vi "(Riemann) Zeta Function.vi"(3 "x":cdb) -> (1 "z(x)":cdb)   [LabVIEW 2014, in "NI_Gmath.lvlib"]
doc: "Computes the zeta function."
uses:
  NI_Gmath.lvlib
  lvanlys.dll
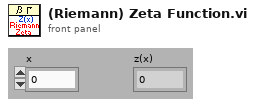
[diagram p1: front panel]
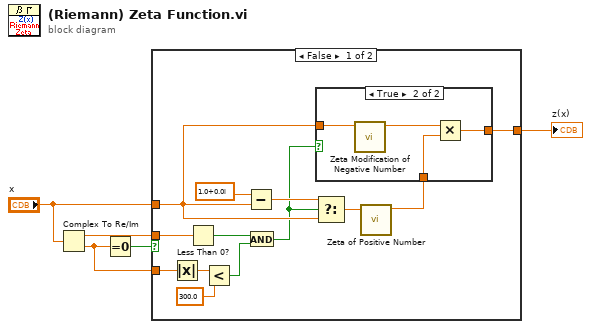
[diagram p0: block diagram]
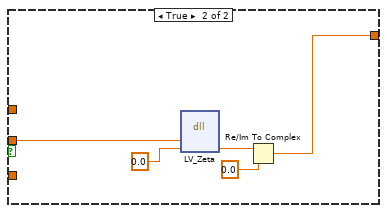
[diagram p3: hidden frame]
diagram:
  n1 = Complex To Re/Im(x + iy="x") -> (x=w5:dbl, y=w3:dbl)
  n2 = Equal To 0?(x=w3) -> (x = 0?=w4:bool)
  n3 = case shown="False" w4 {
    tunnel: "x" -> [w17 _]
    tunnel: w5 -> [w15 w28]
    tunnel: [w16 w25] -> w1
    tunnel: w3 -> [w11 _]
    frame False {
      n4 = Absolute Value(x=w11) -> (abs(x)=w10:dbl)
      n5 = Less Than 0?(x=w15) -> (x < 0?=w7:bool)
      n6 = Less?(x=w10, y=300.0) -> (x < y?=w8:bool)
      n7 = Subtract(x=cdb 1.0+0.0i ("y"), y=w17) -> (x-y=w14:cdb)
      n8 = And(x=w7, y=w8) -> (x .and. y?=w6:bool)
      n9 = Select(t=w14, s=w6, f=w17) -> (s? t:f=w13:cdb)
      n10 = call "Zeta of Positive Number.vi"("x"=w13) -> ("z(x)"=w12:cdb)  [unwired: 9 out]
      n11 = case shown="True" w6 {
        tunnel: w17 -> [_ w21]
        tunnel: w12 -> [w19 w23]
        tunnel: [w19 w22] -> w16
        frame False {
        }
        frame True {
          n12 = call "Zeta Modification of Negative Number.vi"("x"=w21) -> ("r(x)"=w20:cdb)  [unwired: 1 in, 9 out]
          n13 = Multiply(x=w20, y=w23) -> (x*y=w22:cdb)
        }
      }
    }
    frame True {
      n14 = dll-call lib="C:/Program Files (x86)/National Instruments/LabVIEW 2014/resource/lvanlys.*" fn="LV_Zeta"("x"=w28, "Zeta(x)"=0.0 ("y")) -> ("Zeta(x)"=w27:dbl)  [unwired: 4 in, 3 out]
      n15 = Re/Im To Complex(1:0.0 ("y"), 2:w27) -> (0:w25:cdb)
    }
  }
  "z(x)" <- w1
